vi "PiezoSetControlMode.vi"(8 "error in (no error)":errorcluster, 11 "reference":refnum<k7>) -> (0 "error out":errorcluster, 3 "reference out":refnum<k7>)   [LabVIEW 2018]
uses:
  <userlib>/bpc203/PiezoChannelNumber.ctl
  <userlib>/bpc203/PiezoControlMode.ctl
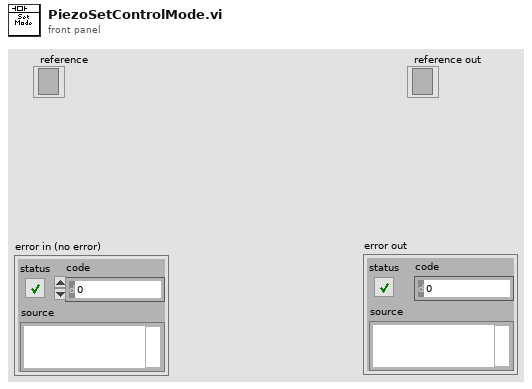
[diagram p1: front panel]
types:
  T1 = typedef "PiezoControlMode.ctl" = u16
  T2 = typedef "PiezoChannelNumber.ctl" = u16
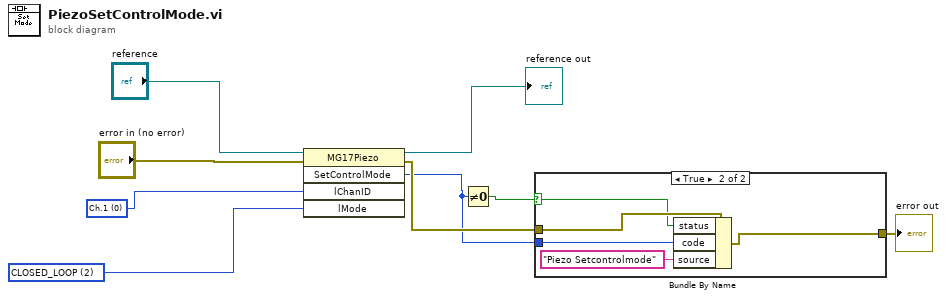
[diagram p0: block diagram]
diagram:
  w3 = T1 2 items=["OPEN_LOOP"=1, "CLOSED_LOOP"=2, "OPEN_LOOP_SMOOTH"=3, "CLOSED_LOOP_SMOOTH"=4, ""=0] ("ctrl_mode")
  w1 = T2 0 items=["Ch.1", "Ch.2"] ("lChanID")
  n1 = invoke class="MG17Piezo" method="SetControlMode"(reference="reference", error in="error in (no error)", "lChanID"=w1, "lMode"=w3) -> (reference out=→"reference out":refnum<k7>, error out=w5:errorcluster, "SetControlMode"=w2:i32)  [unwired: 1 in, 2 out]
  n2 = Not Equal To 0?(x=w2) -> (x != 0?=w6:bool)
  n3 = case shown="True" w6 {
    selector: w6 -> [_ w14]
    tunnel: w5 -> [w10 w15]
    tunnel: [w10 w12] -> w4
    tunnel: w2 -> [_ w11]
    frame False {
    }
    frame True {
      n4 = Bundle By Name(cluster=w15, "status"=w14, "code"=w11, "source"="Piezo Setcontrolmode") -> (w12:errorcluster)
    }
  }
  "error out" <- w4
